vi "Test Handle LogRecord.vi"(8 "error in":errorcluster) -> (0 "error out":errorcluster)   [LabVIEW 2016, in "UT_FileHandler.lvlib"]
doc: "Test the processing of an LogRecord."
uses:
  UT_FileHandler.lvlib
  Source/HSE-Logger/LogLevel.ctl
  Source/HSE-Logger/LogRecord/LogRecord.lvclass/LogRecord.ctl
  Source/HSE-Logger/Handler/FileHandler/FileHandler.lvclass
  <vilib>/addons/_JKI Toolkits/Caraya/classes/Test/Test.lvclass
  Source/HSE-Logger/hse-logger.lvlib
  Source/HSE-Logger/LogRecord/LogRecord.lvclass
  <vilib>/addons/_JKI Toolkits/Caraya/classes/Assert/Assert.lvclass
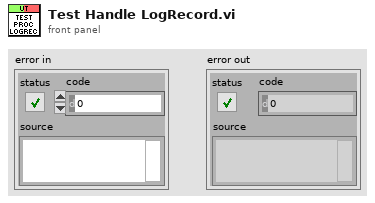
[diagram p1: front panel]
types:
  T1 = typedef "hse-logger.lvlib/LogLevel.ctl" = enum16{"DEBUG", "INFO", "WARNING", "ERROR", "CRITICAL"}
  T2 = enum16{"open", "replace", "create", "open or create", "replace or create", "replace or create with confirmation"}
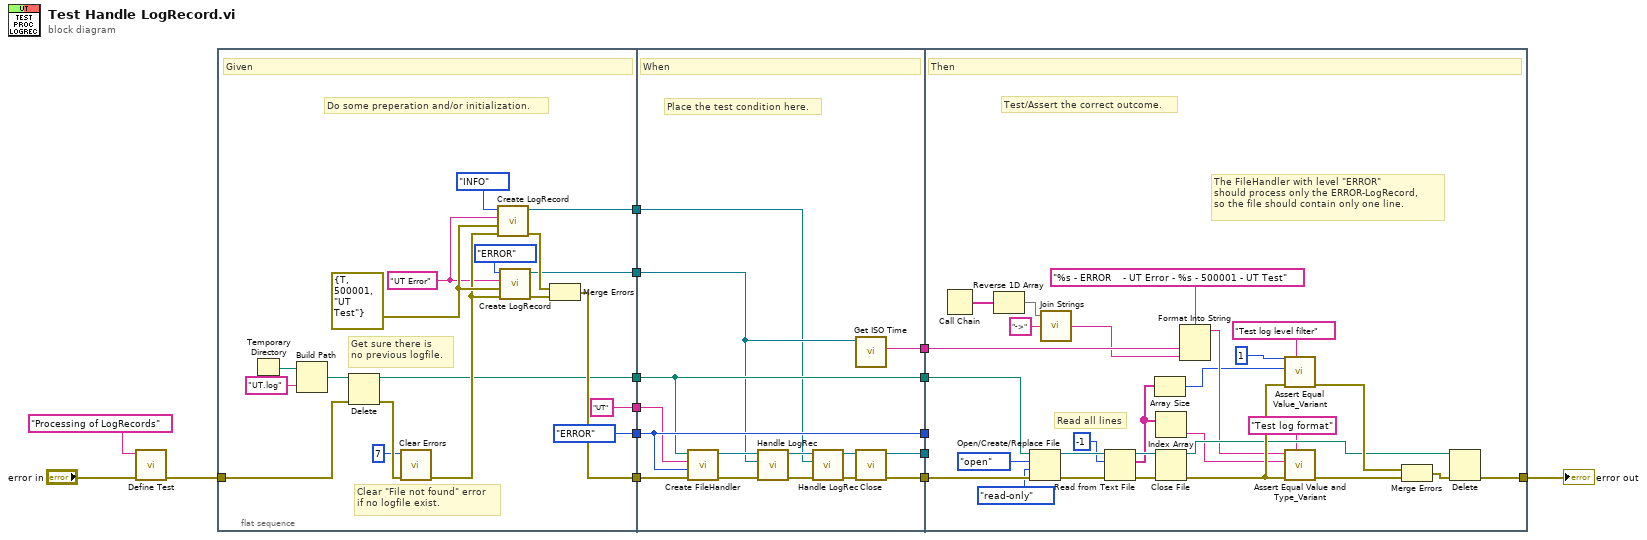
[diagram p0: block diagram]
diagram:
  n1 = call <vilib>:"Define Test.vi"("error in (no error)"="error in", "Label (VI Title)"="Processing of LogRecords") -> ("error out"=w12:errorcluster)  [unwired: 8 in, 1 out]
  n2 = flat-sequence {
    tunnel: w12 -> [w34]
    tunnel: [w29] -> w15
    tunnel: [LogLevel."ERROR" ("Level")] -> w9
    tunnel: ["UT" ("Name")] -> w8
    tunnel: [w22] -> w7
    tunnel: [w19] -> w3
    tunnel: [w17] -> w1
    tunnel: w15 -> [w49]
    tunnel: [w47] -> w11
    tunnel: w9 -> [w44]
    tunnel: w8 -> [w43]
    tunnel: w7 -> [w42]
    tunnel: [w40] -> w6
    tunnel: [w44] -> w5
    tunnel: [w42] -> w4
    tunnel: w3 -> [w39]
    tunnel: [w38] -> w2
    tunnel: w1 -> [w35]
    tunnel: [w71] -> w14
    tunnel: w11 -> [w76]
    tunnel: w6 -> [_]
    tunnel: w5 -> [_]
    tunnel: w4 -> [w69]
    tunnel: w2 -> [w61]
    frame #0 {
      w31 = errorcluster {"status"=TRUE, "code"=500001, "source"="UT Test"} ("Error to Log")
      w18 = "UT Error" ("Message")
      # "Clear \"File not found\" error\nif no logfile exist."
      # "Get sure there is\nno previous logfile."
      # "Do some preperation and/or initialization."
      # "Given"
      n3 = Temporary Directory() -> (w25:path)
      n4 = Build Path(base path=w25, name or relative path="UT.log") -> (appended path=w23:path)
      n5 = Delete(path (use dialog)=w23, error in=w34) -> (deleted path=w22:path, error out=w33:errorcluster)  [unwired: 3 in, 1 out]
      n6 = call <vilib>:"Clear Errors.vi"("error in (no error)"=w33, "specific error code to clear (0: all)"=7) -> ("error out"=w30:errorcluster)  [unwired: 4 in, 1 out]
      n7 = call "Create LogRecord.vi"("error in"=w30, "Error to Log"=w31, "Message"=w18, "Level"=LogLevel."INFO") -> ("error out"=w28:errorcluster, "LogRecord out"=w17:refnum<class "LogRecord.lvclass">)  [unwired: 6 in]
      n8 = call "Create LogRecord.vi"("error in"=w30, "Error to Log"=w31, "Message"=w18, "Level"=LogLevel."ERROR") -> ("error out"=w32:errorcluster, "LogRecord out"=w19:refnum<class "LogRecord.lvclass">)  [unwired: 6 in]
      n9 = Merge Errors(w28, w32) -> (w29:errorcluster)
    }
    frame #1 {
      # "Place the test condition here."
      # "When"
      n10 = call "Create FileHandler.vi"("error in"=w49, "Level"=w44, "Name"=w43, "Filepath"=w42) -> ("error out"=w48:errorcluster, "FileHandler out"=w41:refnum<class "FileHandler.lvclass">)  [unwired: 6 in]
      n11 = call-dynamic "Handle LogRec.vi"("error in"=w48, "LogRecord"=w39, "FileHandler in"=w41) -> ("error out"=w46:errorcluster, "FileHandler out"=w37:refnum<class "FileHandler.lvclass">)  [unwired: 7 in]
      n12 = call-dynamic "Handle LogRec.vi"("error in"=w46, "LogRecord"=w35, "FileHandler in"=w37) -> ("error out"=w45:errorcluster, "FileHandler out"=w36:refnum<class "FileHandler.lvclass">)  [unwired: 7 in]
      n13 = call "Get ISO Time.vi"("LogRecord in"=w39) -> ("ISO Time"=w38:string)  [unwired: 8 in, 2 out]
      n14 = call-dynamic "Close.vi"("error in"=w45, "FileHandler in"=w36) -> ("error out"=w47:errorcluster, "FileHandler out"=w40:refnum<class "FileHandler.lvclass">)  [unwired: 8 in]
    }
    frame #2 {
      # "The FileHandler with level \"ERROR\"\nshould process only the ERROR-LogRecord,\nso the file should contain only one line."
      # "Read all lines"
      # "Test/Assert the correct outcome."
      # "Then"
      n15 = Call Chain() -> (call chain=w51:string[])
      n16 = Reverse 1D Array(array=w51) -> (reversed array=w50:string[])
      n17 = Open/Create/Replace File(file path (use dialog)=w69, error in=w76, operation (0:open)=T2."open", access (0:read/write)=enum16{"read/write", "read-only", "write-only"}."read-only") -> (refnum out=w66:refnum<file>, error out=w75:errorcluster)  [unwired: 2 in, 1 out]
      n18 = call <vilib>:"Join Strings.vi"("Separator (,)"="->", "Strings In"=w50) -> ("String"=w52:string)  [unwired: 1 in]
      n19 = Read from Text File(file (use dialog)=w66, count=-1, error in=w75) -> (refnum out=w65:refnum<file>, text=w58:string[], error out=w73:errorcluster)  [unwired: 1 in, 1 out]
      n20 = Array Size(array=w58) -> (size(s)=w56:i32)
      n21 = Index Array(array=w58) -> (element=w59:string)  [unwired: 1 in]
      n22 = Close File(refnum=w65, error in=w73) -> (path=w64:path, error out=w70:errorcluster)
      n23 = Format Into String(format string="%s - ERROR    - UT Error - %s - 500001 - UT Test" ("text"), w61, w52) -> (resulting string=w62:string)  [unwired: 2 in, 1 out]
      n24 = call <vilib>:"Assert Equal Value_Variant.vi"("Label"="Test log level filter", "error in (no error)"=w70, "Y"=w56, "X"=1 ("size(s)")) -> ("error out"=w77:errorcluster)  [unwired: 6 in, 1 out]
      n25 = call <vilib>:"Assert Equal Value and Type_Variant.vi"("Label"="Test log format", "error in (no error)"=w70, "Y"=w59, "X"=w62) -> ("error out"=w74:errorcluster)  [unwired: 6 in, 1 out]
      n26 = Merge Errors(w77, w74) -> (w72:errorcluster)
      n27 = Delete(path (use dialog)=w64, error in=w72) -> (error out=w71:errorcluster)  [unwired: 3 in, 2 out]
    }
  }
  "error out" <- w14
